vi "Write Comm State.vi"(8 "error in (no error)":errorcluster, 11 "NI-XNET in":refnum<class "NI-XNET.lvclass">) -> (0 "error out":errorcluster, 3 "NI-XNET out":refnum<class "NI-XNET.lvclass">)   [LabVIEW 2023, in "HardwareAbstractionLayer_LVOOP.lvlib" / "CAN HAL Lib.lvlib" / "NI-XNET.lvclass"]
uses:
  NI-XNET.lvclass
  NI-XNET.lvclass/NI-XNET.ctl
  <vilib>/xnet/xnet.llb/XNET Read (State CAN Comm).vi
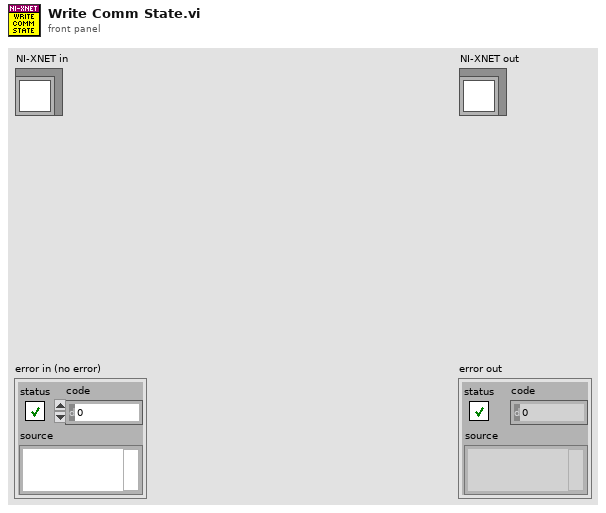
[diagram p1: front panel]
types:
  T1 = typedef "XNET CAN Comm.ctl" = cluster{"fault code":i32, "fault?":bool, "communication state":T2, "last error":T3, "receive error counter":u8, "transmit error counter":u8, "transceiver error?":bool, "sleep?":bool}
  T2 = typedef "XNET CAN Comm State.ctl" = u8
  T3 = typedef "XNET CAN Last Err.ctl" = u8
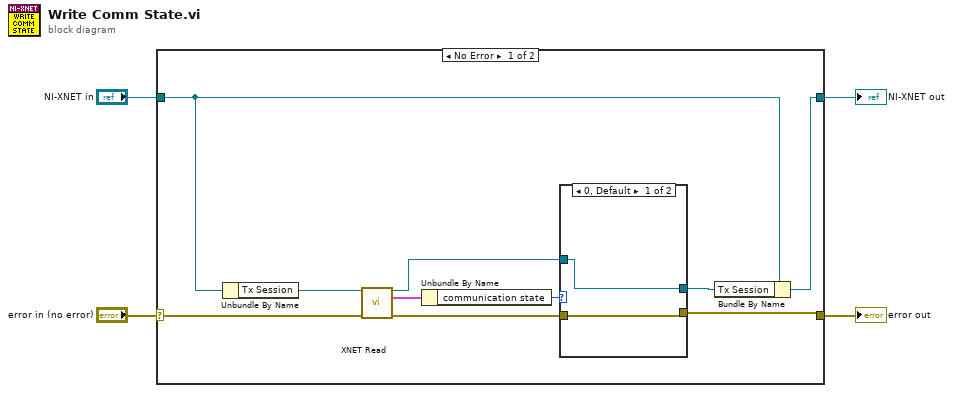
[diagram p0: block diagram]
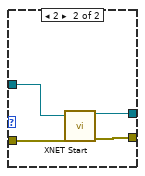
[diagram p2: hidden frame]
diagram:
  n1 = case shown="No Error" "error in (no error)" {
    selector: "error in (no error)" -> [w13 w22]
    tunnel: "NI-XNET in" -> [w7 w21]
    tunnel: [w9 w22] -> w2
    tunnel: [w5 w21] -> w1
    frame No Error {
      n2 = Unbundle By Name(w7) -> ("Tx Session"=w14:refnum<k21>)
      n3 = call-poly <vilib>:"XNET Read.vi"("session in"=w14, "error in (no error)"=w13) -> ("session out"=w8:refnum<k21>, "CAN comm"=w11:T1, "error out"=w12:errorcluster)  [unwired: 11 in]
      n4 = Unbundle By Name(w11) -> ("communication state"=w10:T2)
      n5 = case shown="0, Default" w10 {
        tunnel: w12 -> [w16 w19]
        tunnel: [w16 w20] -> w9
        tunnel: w8 -> [w15 w18]
        tunnel: [w15 w17] -> w6
        frame 0, Default {
        }
        frame 2 {
          n6 = call <vilib>:"XNET Start.vi"("session in"=w18, "error in (no error)"=w19) -> ("session out"=w17:refnum<k21>, "error out"=w20:errorcluster)  [unwired: 12 in]
        }
      }
      n7 = Bundle By Name(cluster=w7, "Tx Session"=w6) -> (w5:refnum<class "NI-XNET.lvclass">)
    }
    frame Error {
    }
  }
  "error out" <- w2
  "NI-XNET out" <- w1
